vi "Main_180803.vi"() -> ()   [LabVIEW 2017, in "Retrieved Data.lvclass"]
uses:
  Retrieved Data.lvclass
  <vilib>/Utility/config.llb/Config Data RefNum.ctl
  <vilib>/Utility/sysdir.llb/System Directory Type.ctl
  <vilib>/Utility/miscctls.llb/LVRowAndColumnTypeDef.ctl
  <vilib>/Utility/file.llb/Write Delimited Spreadsheet (string).vi
  <vilib>/Analysis/NI_AALPro.lvlib
  <vilib>/Utility/config.llb/NI_LVConfig.lvlib
  C:/Users/KimYG/Application/Solution Package/Minhee Retriever/binaries/Microsoft.WindowsAPICodePack.Shell.dll
  binaries/Microsoft.WindowsAPICodePack.Shell.dll
panel:
  in  "ExplorerBrowser":refnum<k24>(container)
  out "StateFileRefnum":T1
  in  "Address":string="C:\\Users\\KimYG\\Application\\Solution Package"
  in  "Retrieved Data.lvclass":refnum<class "Retrieved Data.lvclass">
  in  "Reset":bool caption="Open"
  in  "Copy to Clipboard":bool caption="Blank"
  in  "Comparison":bool caption="Stop"
  in  "Open in file explorer":bool
  in  "Info":bool
  in  "Folders to Exclude":string[](array[string]) caption="Folders to exclude"
  in  "Load":bool
  in  "Save":bool caption="Stop"
  in  "Stop":bool
  in  "Pattern":string="??????_B6_SC_#??.txt"
  in  "Folder Path":path=path "C:/Users/KimYG/Desktop" caption="Data File folder 경로"
  in  "Multicol listbox":i32(listbox)
  out "Query result":string[][](table)
  in  "Significant level (t-test)":enum16{"0.05", "0.01"}(ring)
  in  "Number of bin":dbl=500.0
  in  "Significant level":enum16{"0.05", "0.01"}(ring)
  in  "Data-set II":u16(ring) items=["??????_B6_VC_#??.txt"]
  in  "Data-set I":u16(ring) items=["??????_B6_VC_#??.txt"]
  out "IEI":T2(graph) caption="히스토그램 그래프"
  out "Amplitude":T2(graph) caption="히스토그램 그래프"
  out "P <":dbl format="%#_4g"
  out "P <":dbl format="%#_4g"
  out "P-value":dbl format="%#_4g"
  out "P-value":dbl format="%#_4g"
  out "Mean frequency":cluster{dbl[], dbl[]}[](graph)
  out "Mean amplitude":cluster{dbl[], dbl[]}[](graph)
  out "CP_IEI":cluster{"X Values":dbl[], dbl[]}[](graph) caption="히스토그램 그래프"
  out "CP_Amplitude":cluster{"X Values":dbl[], dbl[]}[](graph) caption="히스토그램 그래프"
  # "Minhee Retriever ver. 1.00 (18.07.11)"
  # "Comparison analysis parameter"
  # "t-test"
  # "K-S test"
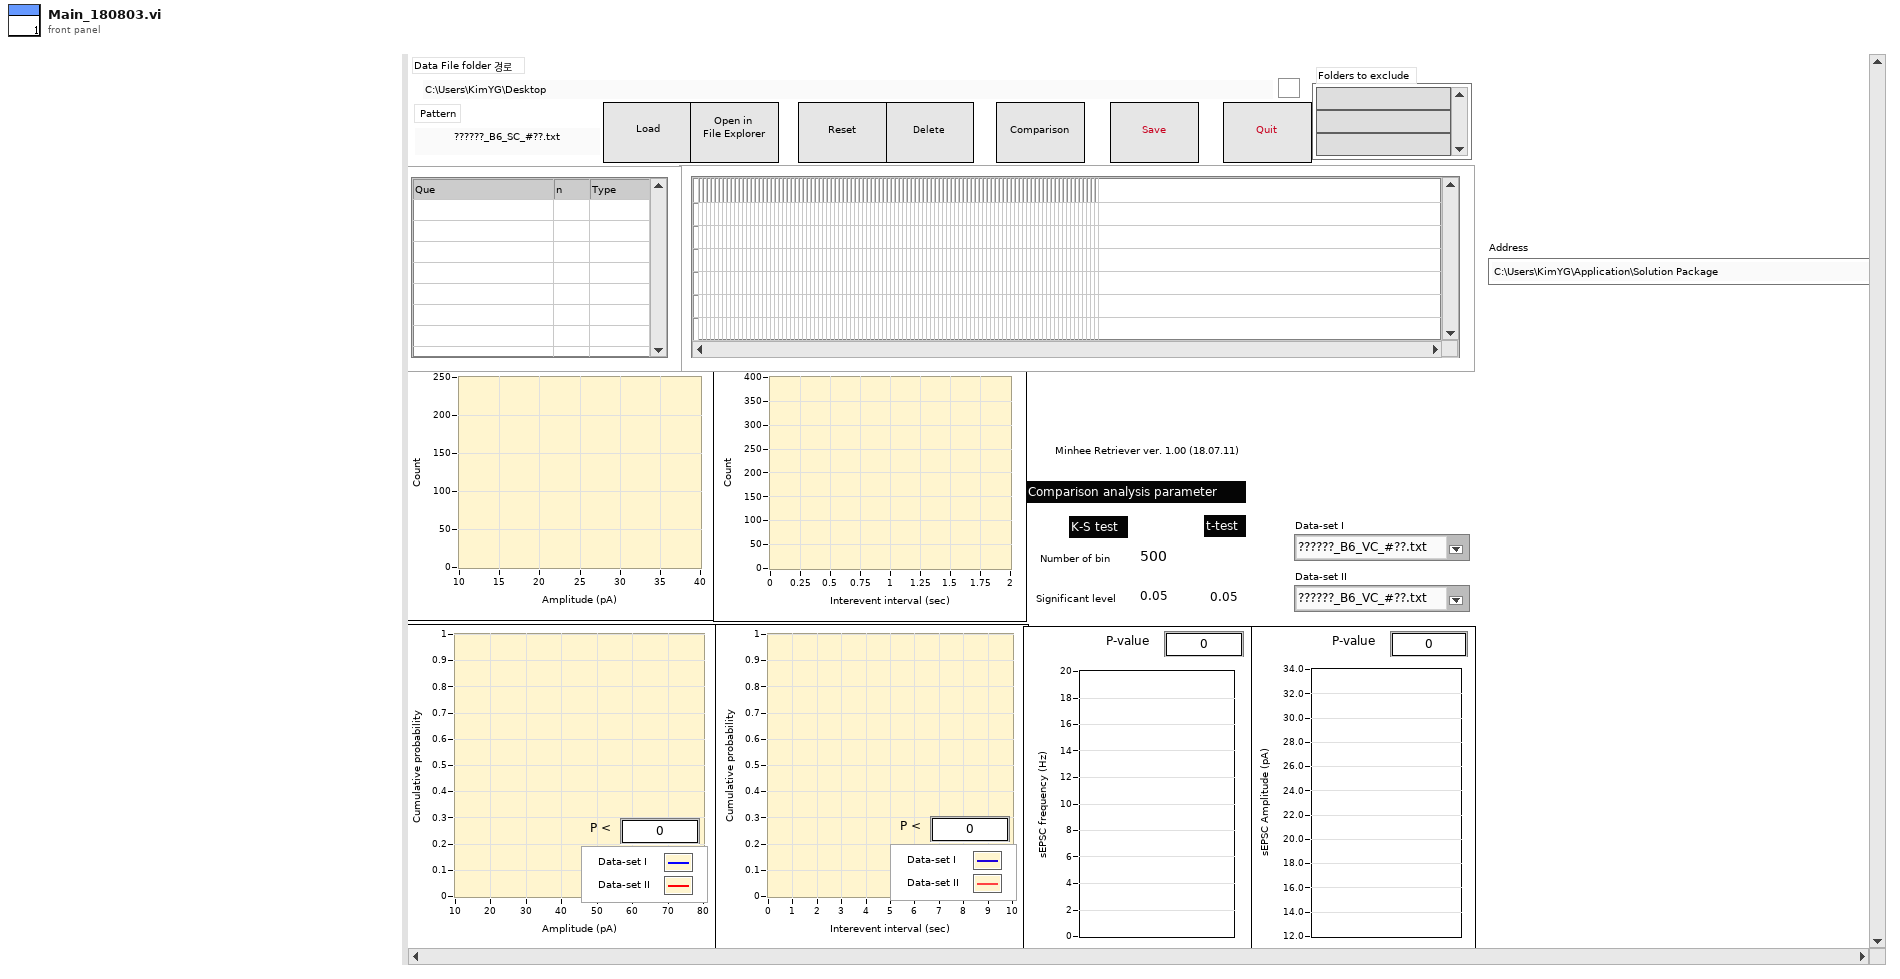
[diagram p1: front panel]
types:
  T1 = typedef "NI_LVConfig.lvlib/Config Data RefNum.ctl" = refnum<k1>
  T2 = cluster{"X Values":dbl[], "Histogram: h(x)":i32[]}
  T3 = typedef "LVRowAndColumnTypeDef.ctl" = cluster{"Row":i32, "Column":i32}
  T4 = typedef "System Directory Type.ctl" = i32
  T5 = cluster{"Que":string, "File name":string[], "Summary":string[][], "Input + Mean,SD,SEM":dbl[][], "Amplitude (pA)":dbl[], "IEI (sec)":dbl[], "Colnames":string[], "Rownames":string[]}
  T6 = cluster{"Folder Path":path, "Pattern":string, "Folders to Exclude":string[]}
  T7 = cluster{"Data-set I":u16, "Data-set II":u16, "Significant level":enum16{"0.05", "0.01"}, "Number of bin":dbl, "Significant level (t-test)":enum16{"0.05", "0.01"}}
  T8 = typedef "Comparison OUT.ctl" = cluster{"CP_Amplitude":cluster{"X Values":dbl[], dbl[]}[], "CP_IEI":cluster{"X Values":dbl[], dbl[]}[], "Mean Amplitude":cluster{dbl[], dbl[]}[], "Mean frequency":cluster{dbl[], dbl[]}[], "t-statistics":cluster{"t-Value":dbl, "DF":i32, "P-value":dbl}[], "KS statistics":cluster{"D":dbl, "Z":dbl, "Reject null hypothesis":bool, "P <":dbl}[]}
  T9 = cluster{"t-Value":dbl, "DF":i32, "P-value":dbl}[]
  T10 = cluster{"D":dbl, "Z":dbl, "Reject null hypothesis":bool, "P <":dbl}[]
  T11 = cluster{"D":dbl, "Z":dbl, "Reject null hypothesis":bool, "P <":dbl}
  T12 = enum32{"invalid app kind", "Development System", "Run Time System", "Student Edition", "Embedded LabVIEW", "Evaluation", "Custom"}
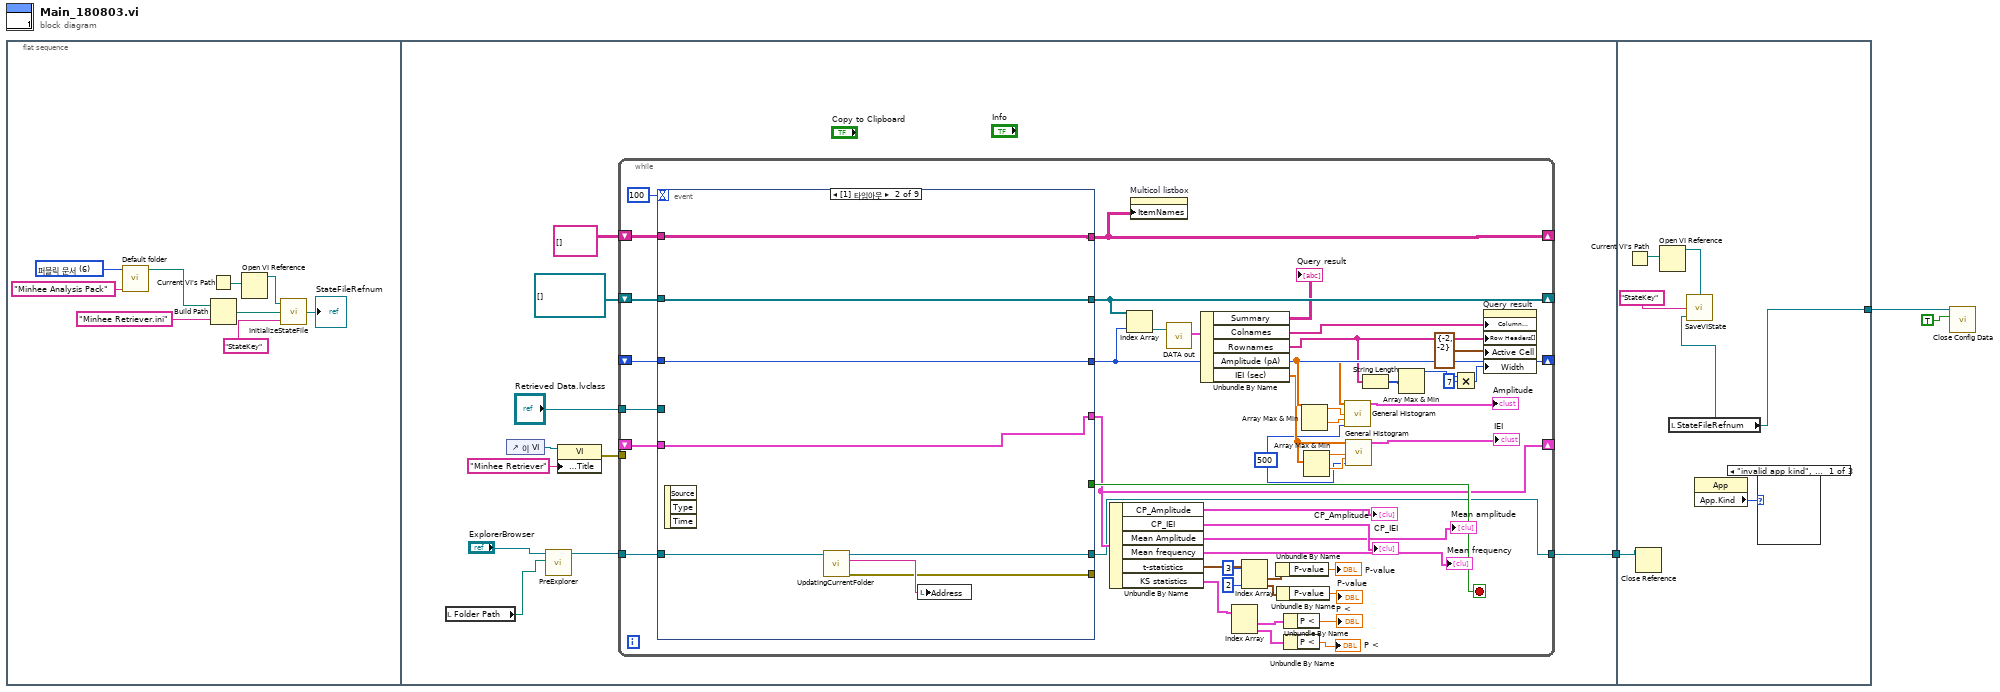
[diagram p0: block diagram]
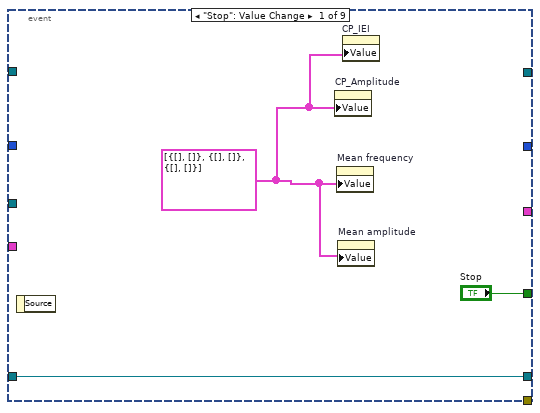
[diagram p2: hidden frame]
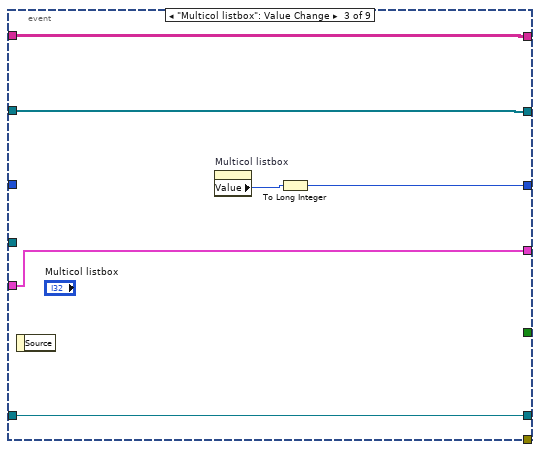
[diagram p3: hidden frame]
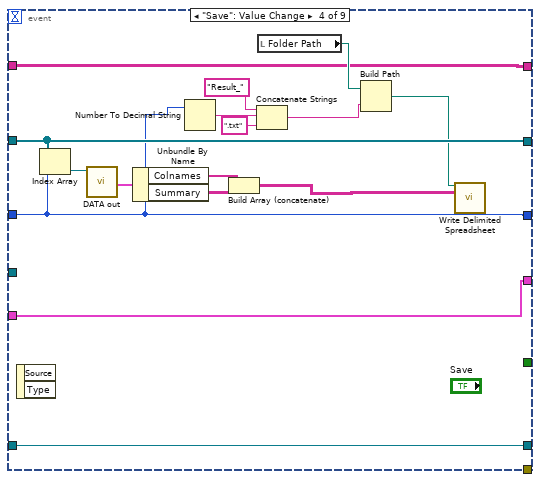
[diagram p4: hidden frame]
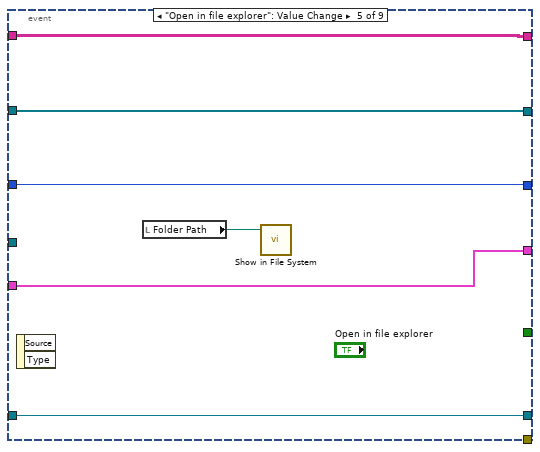
[diagram p5: hidden frame]
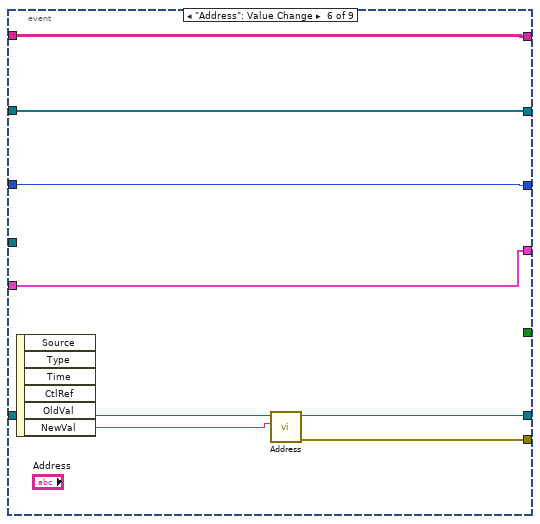
[diagram p6: hidden frame]
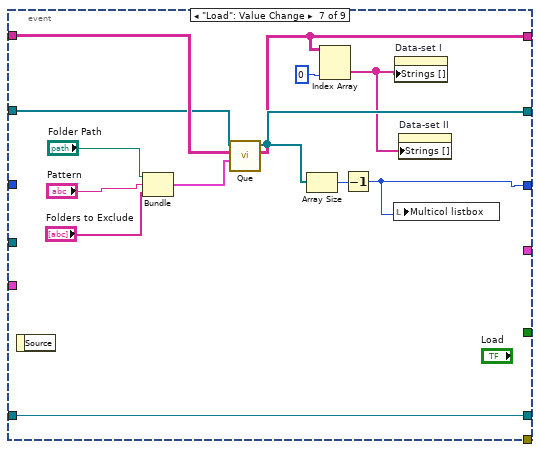
[diagram p7: hidden frame]
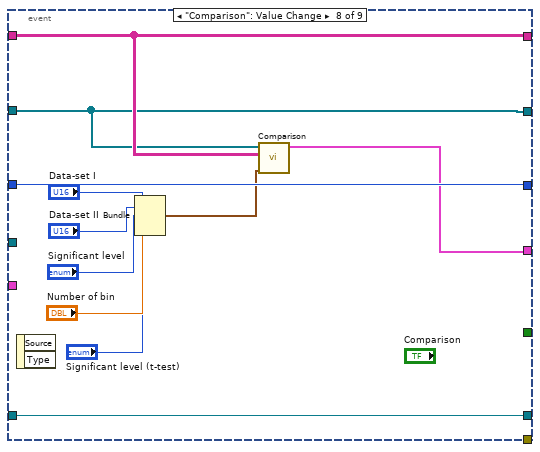
[diagram p8: hidden frame]
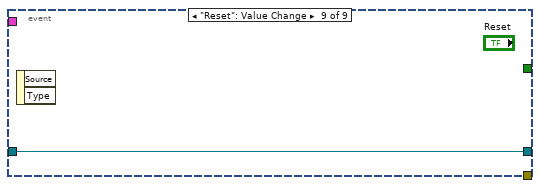
[diagram p9: hidden frame]
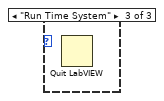
[diagram p11: hidden frame]
diagram:
  n1 = flat-sequence {
    tunnel: [w14] -> w1
    tunnel: [w144] -> w2
    tunnel: w1 -> [w143]
    frame #0 {
      w10 = T4 6 items=["사용자 홈"=0, "사용자 데스크탑"=1, "사용자 문서"=2, "사용자 어플리케이션 데이터"=3, "사용자 환경"=4, "사용자 임시"=5, "퍼블릭 문서"=6, "퍼블릭 어플리케이션 데이터"=7, "퍼블릭 환경"=8, "퍼블릭 캐시"=13, "시스템 코어 라이브러리"=9, "시스템 설치된 라이브러리"=10, "어플리케이션 파일"=11, "부팅 볼륨 루트"=12] ("system directory type")
      n2 = call <userlib>:"Default folder.vi"("Folder name"="Minhee Analysis Pack", "system directory type"=w10) -> ("Folder path"=w12:path)  [unwired: 5 in]
      n3 = Current VI's Path ("Current VI Path...")() -> (path=w8:path)
      n4 = Build Path(base path=w12, name or relative path="Minhee Retriever.ini") -> (appended path=w4:path)
      n5 = Open VI Reference(vi path=w8) -> (vi reference=w7:refnum<vi>)  [unwired: 5 in, 1 out]
      n6 = call <userlib>:"InitializeStateFile.vi"("key"="StateKey", "configuration file path"=w4, "VI Refnum"=w7) -> ("StateFileRefnum"=→"StateFileRefnum":T1)
    }
    frame #1 {
      n7 = local read "Folder Path"() -> (w13:path)
      n8 = control-ref of="이 VI"() -> (w19:refnum<vi>)
      n9 = call "PreExplorer.vi"("Application Directory"=w13, ".NET 참조 번호 입력"="ExplorerBrowser") -> (".NET 참조 번호 출력"=w15:refnum<k24>)  [unwired: 8 in, 1 out]
      n10 = property class="VI"(reference=w19, "Front Panel.Title"="Minhee Retriever" ("프런트패널 윈도우:제목")) -> (error out=w17:errorcluster)  [unwired: 1 in, 1 out]
      n11 = while {
        shift-right: [w68] -> _
        shift-left: string[][] [] -> [w69]
        shift-right: [w65] -> _
        shift-left: refnum<class "Retrieved Data.lvclass">[] [] -> [w67]
        shift-right: [w64] -> _
        shift-left: _ -> [w66]
        tunnel: "Retrieved Data.lvclass" -> [w62]
        tunnel: w17 -> [_]
        shift-right: [w31] -> _
        shift-left: _ -> [w49]
        tunnel: w15 -> [w24]
        tunnel: [w25] -> w14
        stop <- w70 stop-if-true
        w50 = 500 ("# bins")
        n12 = event shown="[1] 타임아웃" {
          selector: _ -> [_ _ _ _ _ _ _ _ _]
          dyn-events: _ -> [_ _ _ _ _ _ _ _ _]
          timeout: 100 -> [_ _ _ _ _ _ _ _ _]
          tunnel: ["Stop" _ _ _ _ _ _ _ _] -> w70
          tunnel: w69 -> [_ w77 w87 w95 w108 w113 w124 w140 _]
          tunnel: [_ w77 w87 w95 w108 w113 w120 w140 _] -> w68
          tunnel: w67 -> [_ w76 w84 w102 w109 w112 w123 w139 _]
          tunnel: [_ w76 w84 w102 w109 w112 w122 w139 _] -> w65
          tunnel: [_ w75 w85 w93 w107 w111 w125 w141 _] -> w64
          tunnel: w66 -> [_ w75 _ w93 w107 w111 _ w141 _]
          tunnel: w62 -> [_ _ _ _ _ _ _ _ _]
          tunnel: [_ w74 w83 w103 w106 w110 _ w133 _] -> w31
          tunnel: w49 -> [_ w74 w83 w103 w106 w110 _ _ _]
          tunnel: [w71 w80 w82 w88 w104 w116 w118 w131 w142] -> w25
          tunnel: [_ w78 _ _ _ w115 _ _ _] -> _
          tunnel: w24 -> [w71 w81 w82 w88 w104 w114 w118 w131 w142]
          event "Stop": Value Change {
            w72 = cluster{dbl[], dbl[]}[] [{[], []}, {[], []}, {[], []}] ("Mean frequency")
            n13 = event-data() -> ()  [unwired: 1 in, 1 out]
            n14 = property on="CP_Amplitude" class="XYGraph (엄격한)"("Value"=w72) -> ()  [unwired: 2 in, 2 out]
            n15 = property on="Mean frequency" class="XYGraph (엄격한)"("Value"=w72) -> ()  [unwired: 2 in, 2 out]
            n16 = property on="Mean amplitude" class="XYGraph (엄격한)"("Value"=w72) -> ()  [unwired: 2 in, 2 out]
            n17 = property on="CP_IEI" class="XYGraph (엄격한)"("Value"=w72) -> ()  [unwired: 2 in, 2 out]
          }
          event Timeout {
            n18 = event-data() -> ()  [unwired: 1 in, 3 out]
            n19 = call "UpdatingCurrentFolder.vi"(".NET 참조 번호 입력"=w81) -> ("에러 출력"=w78:errorcluster, "ParsingName"=w79:string, ".NET 참조 번호 출력"=w80:refnum<k24>)  [unwired: 8 in]
            n20 = local write "Address"(w79) -> ()
          }
          event "Multicol listbox": Value Change {
            n21 = event-data() -> ()  [unwired: 1 in, 1 out]
            n22 = property on="Multicol listbox" class="MCListbox (엄격한)"() -> ("Value"=w86:i32)  [unwired: 2 in, 2 out]
            n23 = To Long Integer(number=w86) -> (32bit integer=w85:i32)
          }
          event "Save": Value Change {
            n24 = event-data() -> ()  [unwired: 1 in, 2 out]
            n25 = Index Array(array=w102, index=w93) -> (element=w101:refnum<class "Retrieved Data.lvclass">)
            n26 = call "DATA out.vi"("Class in"=w101) -> ("Data"=w100:T5)  [unwired: 5 in, 1 out]
            n27 = Unbundle By Name(w100) -> ("Colnames"=w99:string[], "Summary"=w98:string[][])
            n28 = Number To Decimal String(number=w93) -> (decimal integer string=w92:string)  [unwired: 1 in]
            n29 = Build Array (concatenate)(w99, w98) -> (w97:string[][])
            n30 = Concatenate Strings("Result_" ("문자열"), w92, ".txt" ("문자열")) -> (w89:string)
            n31 = local read "Folder Path"() -> (w96:path)
            n32 = Build Path(base path=w96, name or relative path=w89) -> (appended path=w94:path)
            n33 = call-poly <vilib>:"Write Delimited Spreadsheet.vi"("file path (dialog if empty)"=w94, "2D data"=w97) -> ()  [unwired: 12 in, 2 out]
          }
          event "Open in file explorer": Value Change {
            n34 = event-data() -> ()  [unwired: 1 in, 2 out]
            n35 = local read "Folder Path"() -> (w105:path)
            n36 = call <vilib>:"Show in File System.vi"("file or directory path"=w105) -> ()  [unwired: 10 in, 1 out]
          }
          event "Address": Value Change {
            n37 = event-data() -> ("NewVal"=w117:string)  [unwired: 1 in, 5 out]
            n38 = call "Address.vi"("NewVal"=w117, ".NET 참조 번호 입력"=w114) -> ("에러 출력"=w115:errorcluster, ".NET 참조 번호 출력"=w116:refnum<k24>)  [unwired: 8 in]
          }
          event "Load": Value Change {
            n39 = event-data() -> ()  [unwired: 1 in, 1 out]
            n40 = Bundle("Folder Path"="Folder Path", "Pattern"="Pattern", "Folders to Exclude"="Folders to Exclude") -> (w127:T6)  [unwired: 1 in]
            n41 = call "Que.vi"("Que info"=w127, "Muticol listbox in"=w124, "Data stack IN"=w123) -> ("Muticol listbox out"=w120:string[][], "Data stack OUT"=w122:refnum<class "Retrieved Data.lvclass">[])  [unwired: 2 in, 1 out]
            n42 = Array Size(array=w122) -> (size(s)=w126:i32)
            n43 = Index Array(array=w120, index (col)=0 ("비활성화된 인덱스 (열)")) -> (element=w119:string[])  [unwired: 1 in]
            n44 = Decrement(x=w126) -> (x-1=w125:i32)
            n45 = local write "Multicol listbox"(w125) -> ()
            n46 = property on="Data-set I" class="Ring (엄격한)"("Strings []"=w119) -> ()  [unwired: 2 in, 2 out]
            n47 = property on="Data-set II" class="Ring (엄격한)"("Strings []"=w119) -> ()  [unwired: 2 in, 2 out]
          }
          event "Comparison": Value Change {
            n48 = event-data() -> ()  [unwired: 1 in, 2 out]
            n49 = Bundle("Data-set I"="Data-set I", "Data-set II"="Data-set II", "Significant level"="Significant level", "Number of bin"="Number of bin", "Significant level (t-test)"="Significant level (t-test)") -> (w134:T7)  [unwired: 1 in]
            n50 = call "Comparison.vi"("Comparison parameter"=w134, "Muticol listbox IN"=w140, "Data Stack IN"=w139) -> ("Comparison out"=w133:T8)  [unwired: 4 in]
          }
          event "Reset": Value Change {
            n51 = event-data() -> ()  [unwired: 1 in, 2 out]
          }
        }
        n52 = Unbundle By Name(w31) -> ("CP_Amplitude"=→"CP_Amplitude":cluster{"X Values":dbl[], dbl[]}[], "CP_IEI"=→"CP_IEI":cluster{"X Values":dbl[], dbl[]}[], "Mean Amplitude"=→"Mean amplitude":cluster{dbl[], dbl[]}[], "Mean frequency"=→"Mean frequency":cluster{dbl[], dbl[]}[], "t-statistics"=w44:T9, "KS statistics"=w30:T10)
        n53 = Index Array(array=w65, index=w64) -> (element=w63:refnum<class "Retrieved Data.lvclass">)
        n54 = property on="Multicol listbox" class="MCListbox (엄격한)"("ItemNames"=w68) -> ()  [unwired: 2 in, 2 out]
        n55 = call "DATA out.vi"("Class in"=w63) -> ("Data"=w61:T5)  [unwired: 5 in, 1 out]
        n56 = Unbundle By Name(w61) -> ("Summary"=→"Query result":string[][], "Colnames"=w59:string[], "Rownames"=w37:string[], "Amplitude (pA)"=w56:dbl[], "IEI (sec)"=w53:dbl[])
        n57 = Index Array(array=w30) -> (element #1=w29:T11, element #2=w28:T11)  [unwired: 2 in]
        n58 = Index Array(array=w44, index #1=3 ("인덱스"), index #2=2 ("인덱스")) -> (element #1=w43:cluster{"t-Value":dbl, "DF":i32, "P-value":dbl}, element #2=w42:cluster{"t-Value":dbl, "DF":i32, "P-value":dbl})
        n59 = Unbundle By Name(w43) -> ("P-value"=→"P-value":dbl)
        n60 = Unbundle By Name(w42) -> ("P-value"=→"P-value":dbl)
        n61 = Unbundle By Name(w29) -> ("P <"=→"P <":dbl)
        n62 = Unbundle By Name(w28) -> ("P <"=→"P <":dbl)
        n63 = Array Max & Min(array=w56) -> (max value=w54:dbl, min value=w55:dbl)  [unwired: 2 out]
        n64 = Array Max & Min(array=w53) -> (max value=w52:dbl, min value=w51:dbl)  [unwired: 2 out]
        n65 = call <vilib>:"General Histogram.vi"("X"=w56, "max"=w54, "min"=w55, "# bins"=w50) -> ("Histogram Graph"=→"Amplitude":T2)  [unwired: 7 in, 4 out]
        n66 = call <vilib>:"General Histogram.vi"("X"=w53, "max"=w52, "min"=w51, "# bins"=w50) -> ("Histogram Graph"=→"IEI":T2)  [unwired: 7 in, 4 out]
        n67 = String Length(string=w37) -> (length=w36:i32[])
        n68 = Array Max & Min(array=w36) -> (max value=w35:i32)  [unwired: 3 out]
        n69 = Multiply(x=w35, y=7) -> (x*y=w33:i32)
        n70 = property on="Query result" class="Tbl (엄격한)"("Column Headers[]"=w59, "Row Headers[]"=w37, "Active Cell"=T3 {"Row"=-2, "Column"=-2} ("활성 셀:활성 셀"), "Width"=w33) -> ()  [unwired: 2 in, 2 out]
      }
    }
    frame #2 {
      n71 = Current VI's Path ("Current VI's Path...")() -> (path=w146:path)
      n72 = Close Reference(reference=w143) -> ()  [unwired: 1 in, 1 out]
      n73 = Open VI Reference(vi path=w146) -> (vi reference=w147:refnum<vi>)  [unwired: 5 in, 1 out]
      n74 = local read "StateFileRefnum"() -> (w144:T1)
      n75 = call <userlib>:"SaveVIState.vi"("StateFileRefnum"=w144, "key"="StateKey", "VI Refnum"=w147) -> ()
      n76 = property class="App"() -> ("App.Kind"=w145:T12)  [unwired: 2 in, 2 out]
      n77 = case shown="\"invalid app kind\", 기본" w145 {
        frame "invalid app kind", Default {
        }
        frame "Development System" {
        }
        frame "Run Time System" {
          n78 = Quit LabVIEW() -> ()  [unwired: 1 in]
        }
      }
    }
  }
  n79 = call <vilib>:"Close Config Data.vi"("write file if changed (T)"=TRUE ("write configuration file? (F)"), "refnum"=w2) -> ()  [unwired: 8 in, 2 out]
